vi "BuildHWI.vi"(8 "error in (no error)":errorcluster, 10 "Master Device in":refnum<class "Master Device.lvclass">, 11 "Slave_Pulseblaster in":refnum<class "Slave_Pulseblaster.lvclass">) -> (0 "error out":errorcluster, 2 "Master Device out":refnum<class "Master Device.lvclass">, 3 "Slave_Pulseblaster out":refnum<class "Slave_Pulseblaster.lvclass">)   [LabVIEW 2013, in "Slave_Pulseblaster.lvclass"]
doc: "The previous subVI Prune.vi took the \"prepared\" private data and removed unnecessary points. Here in BuildHWI, one should turn the \"prepared\" data into a HWI that can be programmed to the physical device.\n (1) Flatten the data structure and put in normal time order"
uses:
  Slave_Pulseblaster.lvclass
  Device/Device.lvclass
  Master Device/Master Device.lvclass
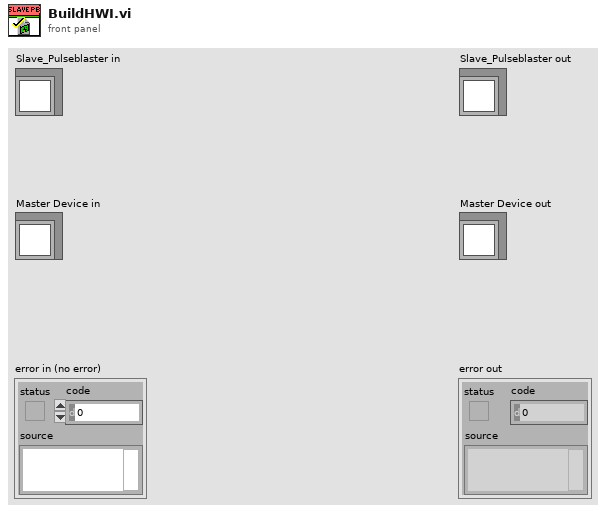
[diagram p1: front panel]
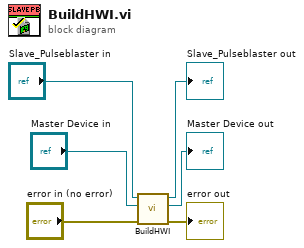
[diagram p0: block diagram]
diagram:
  n1 = call-parent "BuildHWI.vi"("error in (no error)"="error in (no error)", "Master Device in"="Master Device in", "Device in"="Slave_Pulseblaster in") -> ("error out"=→"error out":errorcluster, "Master Device out"=→"Master Device out":refnum<class "Master Device.lvclass">, "Device out"=→"Slave_Pulseblaster out":refnum<class "Slave_Pulseblaster.lvclass">)  [unwired: 6 in]
